vi "action.vi"(0 "NInstrSim_ConfigureWaveformType":refnum<class "NInstrSim_ConfigureWaveformType.lvclass">, 2 "HGF_Visitable":refnum<class "HGF_Visitable.lvclass">, 5 "error in (no error)":errorcluster) -> (14 "dup NInstrSim_ConfigureWaveformType":refnum<class "NInstrSim_ConfigureWaveformType.lvclass">, 16 "dup HGF_Visitable":refnum<class "HGF_Visitable.lvclass">, 19 "error out":errorcluster)   [LabVIEW 2009, in "HB_Device_Examples.lvlib" / "NInstrSim_ConfigureWaveformType.lvclass"]
doc: "This is a dynamic dispatch VI that is called from Visitor.visit(). It will call member VIs of Visitable to perform the requested action which means: calling public methods of Visitable child class.\n\n<B>Hint:</B> This method is abstract and need to be implemented by child classes."
uses:
  NInstrSim_ConfigureWaveformType.lvclass
  lib.lib/HGF_LVC/HGF_BaseClasses/HGF_Visitable/HGF_Visitable.lvclass
  NInstrSim.lvclass
  NInstrSim_ConfigureWaveformType.lvclass/NInstrSim_ConfigureWaveformType.ctl
  lib.lib/HGF_LVC/HGF_BaseClasses/HGF_NetworkVisitor/HGF_NetworkVisitor.lvclass
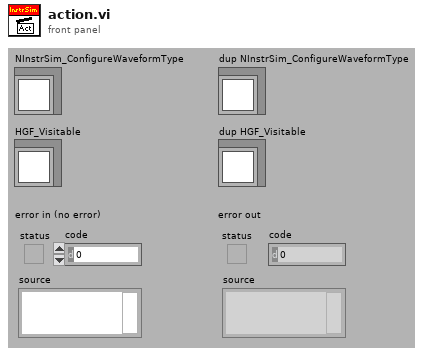
[diagram p1: front panel]
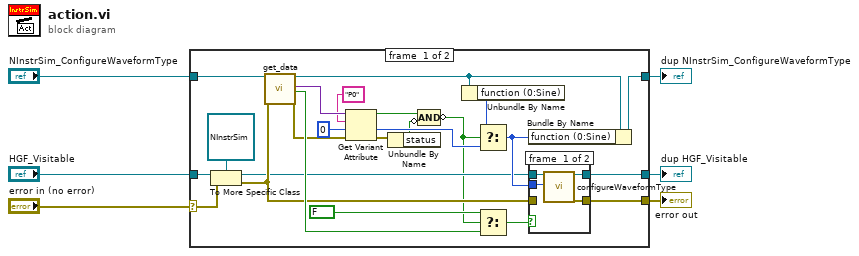
[diagram p0: block diagram]
diagram:
  n1 = case shown="No Error" "error in (no error)" {
    selector: "error in (no error)" -> [w28 w37]
    tunnel: "NInstrSim_ConfigureWaveformType" -> [w17 w39]
    tunnel: "HGF_Visitable" -> [w30 w38]
    tunnel: [w12 w38] -> w4
    tunnel: [w11 w37] -> w3
    tunnel: [w16 w39] -> w1
    frame #0 {
      n2 = To More Specific Class(target class=refnum<class "NInstrSim.lvclass"> refnum ("HB_HGF_Test.lvlib:NInstrSim.lvclass"), reference=w30, error in=w28) -> (specific class reference=w13:refnum<class "NInstrSim.lvclass">, error out=w15:errorcluster)
      n3 = call "get_data.vi"("HGF_NetworkData"=w17, "error in (no error)"=w15) -> ("dup HGF_NetworkData"=w25:refnum<class "NInstrSim_ConfigureWaveformType.lvclass">, "data"=w27:variant, "no link"=w21:bool, "error out"=w14:errorcluster)  [unwired: 14 out]
      n4 = Get Variant Attribute(Variant=w27, name="P0", default value (empty Variant)=u16 0 ("DC Voltage Range (1:10 VDC)"), error in=w14) -> (found=w9:bool, value=w20:u16, error out=w10:errorcluster)  [unwired: 1 out]
      n5 = Unbundle By Name(w10) -> ("status"=w8:bool)
      n6 = Compound Arithmetic op=AND(w9, invert w8) -> (invert w7:bool)
      n7 = Unbundle By Name(w25) -> ("function (0:Sine)"=w22:u16)
      n8 = Select(t=w22, s=w7, f=w20) -> (s? t:f=w26:u16)
      n9 = Select(t=FALSE, s=w7, f=w21) -> (s? t:f=w24:bool)
      n10 = Bundle By Name(cluster=w25, "function (0:Sine)"=w26) -> (w16:refnum<class "NInstrSim_ConfigureWaveformType.lvclass">)
      n11 = case shown="False" w24 {
        tunnel: w13 -> [w32 w36]
        tunnel: [w33 w36] -> w12
        tunnel: [w34 w35] -> w11
        tunnel: w15 -> [_ w35]
        tunnel: w26 -> [w31 _]
        frame #0 {
          n12 = call "configureWaveformType.vi"("NInstrSim"=w32, "function (0:Sine)"=w31) -> ("dup NInstrSim"=w33:refnum<class "NInstrSim.lvclass">, "error out"=w34:errorcluster)  [unwired: 1 in, 15 out]
        }
        frame #1 {
        }
      }
    }
    frame #1 {
    }
  }
  "error out" <- w3
  "dup NInstrSim_ConfigureWaveformType" <- w1
  "dup HGF_Visitable" <- w4
